vi "Event Set Event Raw.vi"(8 "error in (no error)":errorcluster, 9 "Raw data":i8[](array[numeric]), 10 "Event name":string, 11 "Event DVR in":refnum<data-value>) -> (0 "error out":errorcluster, 3 "Event DVR out":refnum<data-value>)   [LabVIEW 2012, in "MDSplus.lvlib"]
doc: "Issues an event passing a simple buffer of bytes (no Data)."
uses:
  <vilib>/MDSplus/Library/MDSplus.lvlib
  <vilib>/MDSplus/Classes/Event_Class/Event.lvclass
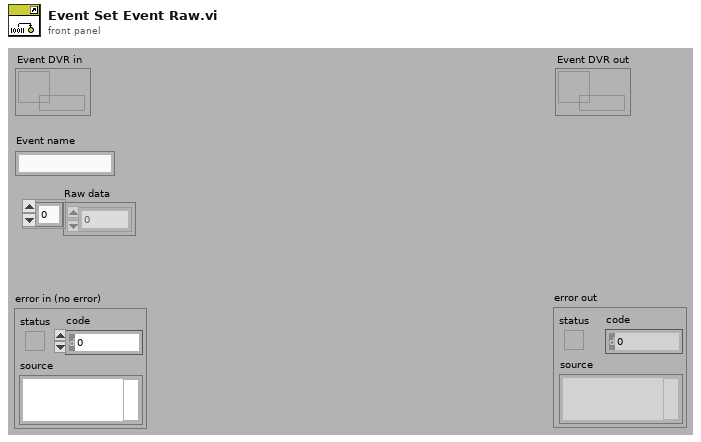
[diagram p1: front panel]
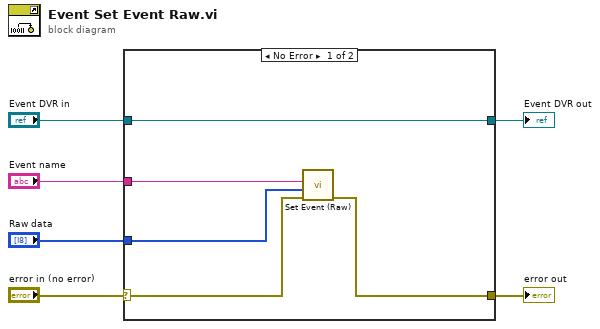
[diagram p0: block diagram]
diagram:
  n1 = case shown="No Error" "error in (no error)" {
    selector: "error in (no error)" -> [w7 w12]
    tunnel: "Event DVR in" -> [w9 w13]
    tunnel: [w10 w12] -> w6
    tunnel: [w9 w13] -> w3
    tunnel: "Event name" -> [w11 _]
    tunnel: "Raw data" -> [w8 _]
    frame No Error {
      n2 = call <vilib>:"Set Event (Raw).vi"("error in (no error)"=w7, "Raw data"=w8, "Event name"=w11) -> ("error out"=w10:errorcluster)  [unwired: 7 in, 1 out]
    }
    frame Error {
    }
  }
  "error out" <- w6
  "Event DVR out" <- w3
